vi "Update Credit.vi"(8 "error in (no error)":errorcluster, 11 "MSG in":refnum<class "MSG.lvclass">) -> (0 "error out":errorcluster, 2 "Credito":dbl, 3 "MSG out":refnum<class "MSG.lvclass">)   [LabVIEW 2020, in "MSG.lvlib" / "MSG.lvclass"]
uses:
  MSG.lvclass
  MSG.lvclass/MSG.ctl
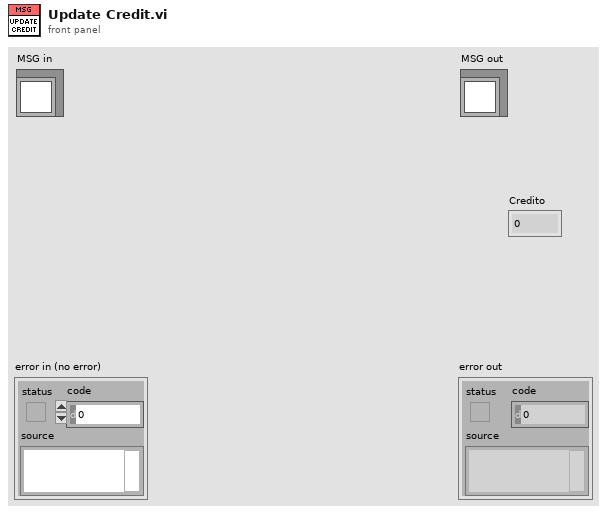
[diagram p1: front panel]
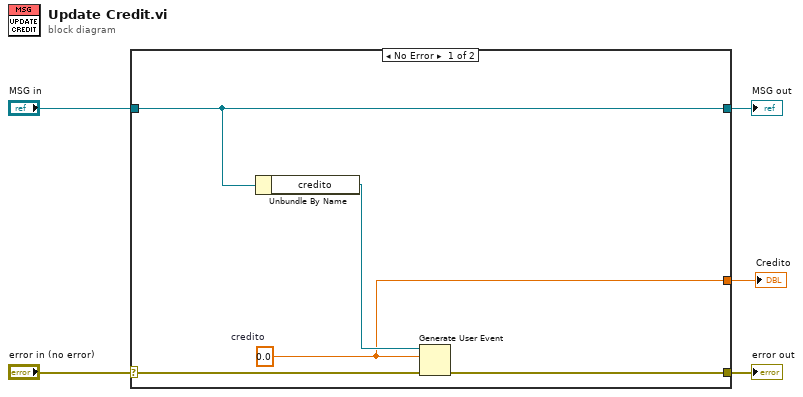
[diagram p0: block diagram]
diagram:
  n1 = case shown="No Error" "error in (no error)" {
    selector: "error in (no error)" -> [w10 w12]
    tunnel: [w8 w12] -> w4
    tunnel: [w9 w11] -> w2
    tunnel: "MSG in" -> [w9 w11]
    tunnel: [w6 _] -> w1
    frame No Error {
      w6 = 0.0  # credito
      n2 = Unbundle By Name(w9) -> ("credito"=w7:refnum<user-event>)
      n3 = Generate User Event(user event=w7, event data cluster=w6, error in=w10) -> (error out=w8:errorcluster)  [unwired: 1 in, 1 out]
    }
    frame Error {
    }
  }
  "error out" <- w4
  "MSG out" <- w2
  "Credito" <- w1
